vi "data_headers 11-08-2017.vi"(10 "Sample names":T1={"QCM1 sample name"="aQCM2", "QCM2 sample name"="aQCM2", "QCM3 sample name"="aQCM3", "QCM4 sample name"="aQCM4", "QCM5 sample name"="aQCM5", "QCM6 sample name"="aQCM6", "SRS sample name"="sample_SRS", "Keithley 2420 sample name"="Keithley2420", "Keithley 6430 sample name"="Keithley6430", "Keithley 2100 sample name"="Keithley6430", "Gas"="aQCM2", "Vapor"="aQCM2", "Experiment Notes"=""}) -> (2 "data headers":string[](array[string]))   [LabVIEW 2014]
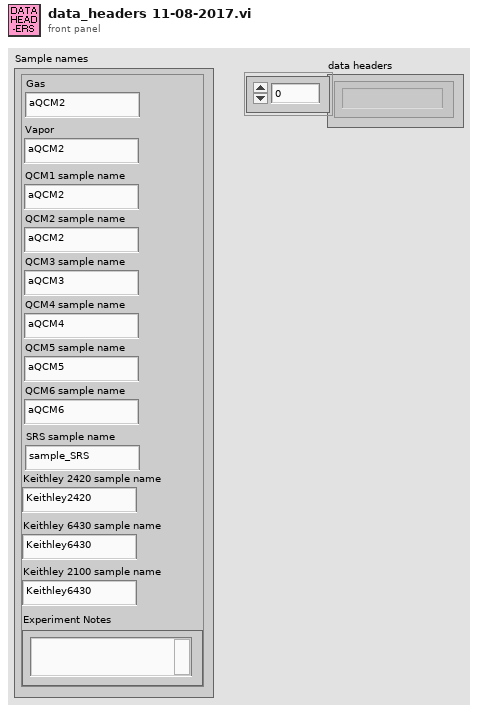
[diagram p1: front panel]
types:
  T1 = cluster{"QCM1 sample name":string, "QCM2 sample name":string, "QCM3 sample name":string, "QCM4 sample name":string, "QCM5 sample name":string, "QCM6 sample name":string, "SRS sample name":string, "Keithley 2420 sample name":string, "Keithley 6430 sample name":string, "Keithley 2100 sample name":string, "Gas":string, "Vapor":string, "Experiment Notes":string}
  T2 = cluster{string, string, string, string, string, string}
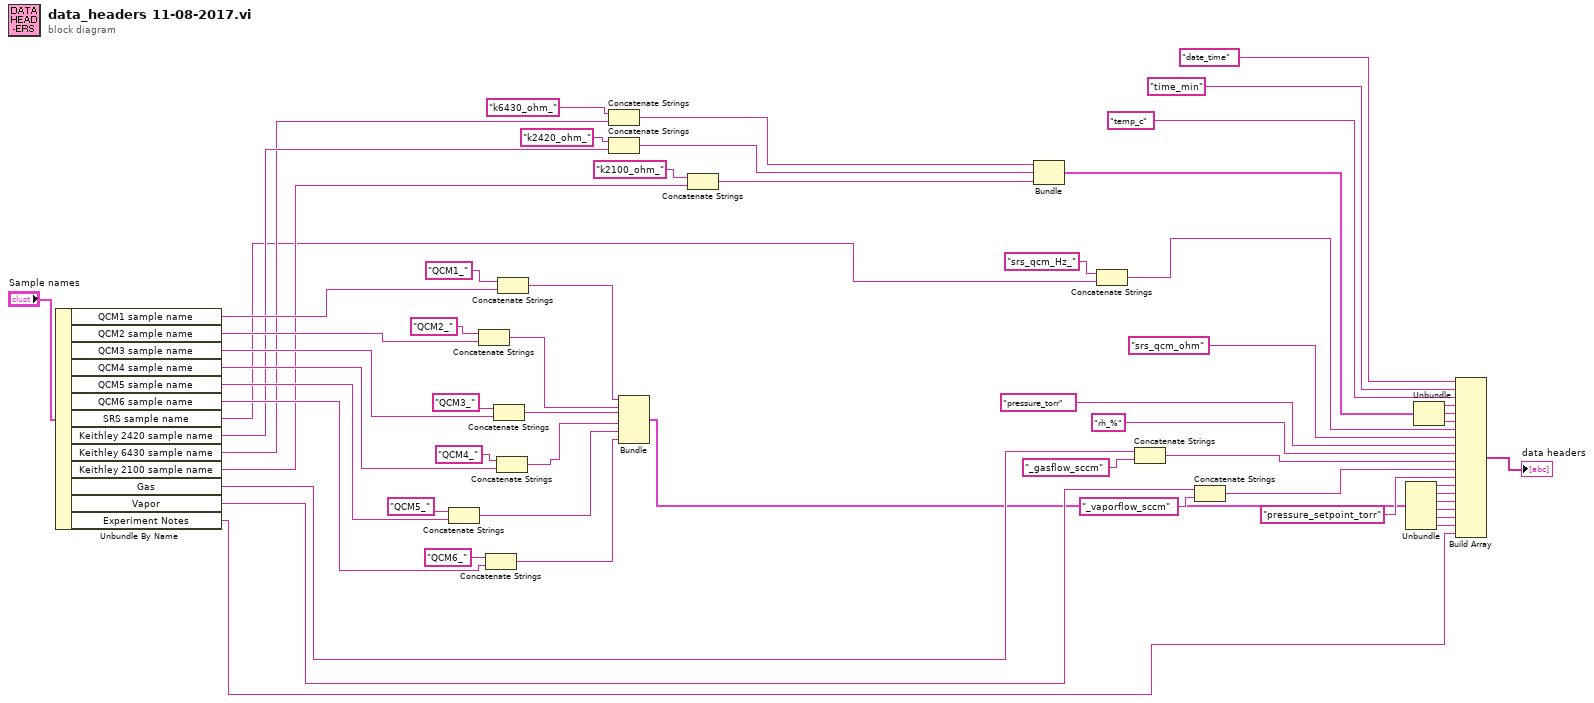
[diagram p0: block diagram]
diagram:
  n1 = Unbundle By Name("Sample names") -> ("QCM1 sample name"=w48:string, "QCM2 sample name"=w45:string, "QCM3 sample name"=w43:string, "QCM4 sample name"=w41:string, "QCM5 sample name"=w38:string, "QCM6 sample name"=w37:string, "SRS sample name"=w3:string, "Keithley 2420 sample name"=w36:string, "Keithley 6430 sample name"=w35:string, "Keithley 2100 sample name"=w33:string, "Gas"=w19:string, "Vapor"=w18:string, "Experiment Notes"=w4:string)
  n2 = Concatenate Strings("QCM5_" ("string"), w38) -> (w13:string)
  n3 = Concatenate Strings("QCM2_" ("string"), w45) -> (w16:string)
  n4 = Concatenate Strings("QCM6_" ("string"), w37) -> (w12:string)
  n5 = Concatenate Strings("QCM3_" ("string"), w43) -> (w15:string)
  n6 = Concatenate Strings("QCM4_" ("string"), w41) -> (w14:string)
  n7 = Concatenate Strings("QCM1_" ("string"), w48) -> (w17:string)
  n8 = Concatenate Strings("k6430_ohm_", w35) -> (w31:string)
  n9 = Concatenate Strings("k2420_ohm_" ("element"), w36) -> (w30:string)
  n10 = Bundle(w17, w16, w15, w14, w13, w12) -> (w11:T2)  [unwired: 1 in]
  n11 = Concatenate Strings("k2100_ohm_" ("element"), w33) -> (w29:string)
  n12 = Bundle(w31, w30, w29) -> (w28:cluster{string, string, string})  [unwired: 1 in]
  n13 = Concatenate Strings("srs_qcm_Hz_", w3) -> (w1:string)
  n14 = Concatenate Strings(w19, "_gasflow_sccm" ("element")) -> (w23:string)
  n15 = Concatenate Strings(w18, "_vaporflow_sccm" ("element")) -> (w22:string)
  n16 = Unbundle(w11) -> (w5:string, w6:string, w7:string, w8:string, w9:string, w10:string)
  n17 = Unbundle(w28) -> (w27:string, w26:string, w25:string)
  n18 = Build Array("date_time", "time_min", "temp_c", w27, w26, w25, w1, "srs_qcm_ohm", "pressure_torr" ("element"), "rh_%" ("element"), w23, w22, "pressure_setpoint_torr" ("element"), w5, w6, w7, w8, w9, w10, w4) -> (→"data headers":string[])
